vi "test-swerve-drive-kinematics-03.vi"() -> (3 "Test Passed":bool)   [LabVIEW 2019]
uses:
  <vilib>/Rock Robotics/WPI/ThirdParty/JAS_Junk/TrajLib/SWERVE_DRIVE_MODULE_STATE.ctl
  <vilib>/Rock Robotics/WPI/ThirdParty/JAS_Junk/TrajLib/ROTATION2D.ctl
  <vilib>/Rock Robotics/WPI/ThirdParty/JAS_Junk/TrajLib/Trajectory_Library.lvlib
panel:
  out "ModuleStates":T1[](array[typedef]) {"Angle"."SIN" format="%13.4f"; "Angle"."COS" format="%13.4f"; "Angle"."VALUE" format="%13.4f"}
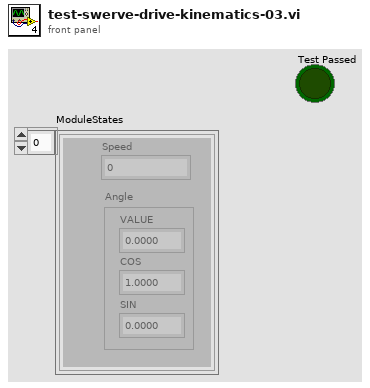
[diagram p1: front panel]
types:
  T1 = typedef "Trajectory_Library.lvlib/SWERVE_DRIVE_MODULE_STATE.ctl" = cluster{"Speed":dbl, "Angle":T2}
  T2 = typedef "Trajectory_Library.lvlib/ROTATION2D.ctl" = cluster{"VALUE":dbl, "COS":dbl, "SIN":dbl}
  T3 = typedef "Trajectory_Library.lvlib/TRANSLATION2D.ctl" = cluster{"X":dbl, "Y":dbl}
  T4 = typedef "Trajectory_Library.lvlib/SWERVE_DRIVE_KINEMATICS.ctl" = cluster{"NumModules":i32, "InverseKinematics":T5, "ForwardKinematics":T5, "Modules":T3[], "PrevCoR":T3}
  T5 = typedef "NI_Matrix.lvlib/RealMatrix.ctl" = dbl[][]
  T6 = typedef "Trajectory_Library.lvlib/CHASSIS_SPEEDS.ctl" = cluster{"vX":dbl, "vY":dbl, "vOmega":dbl}
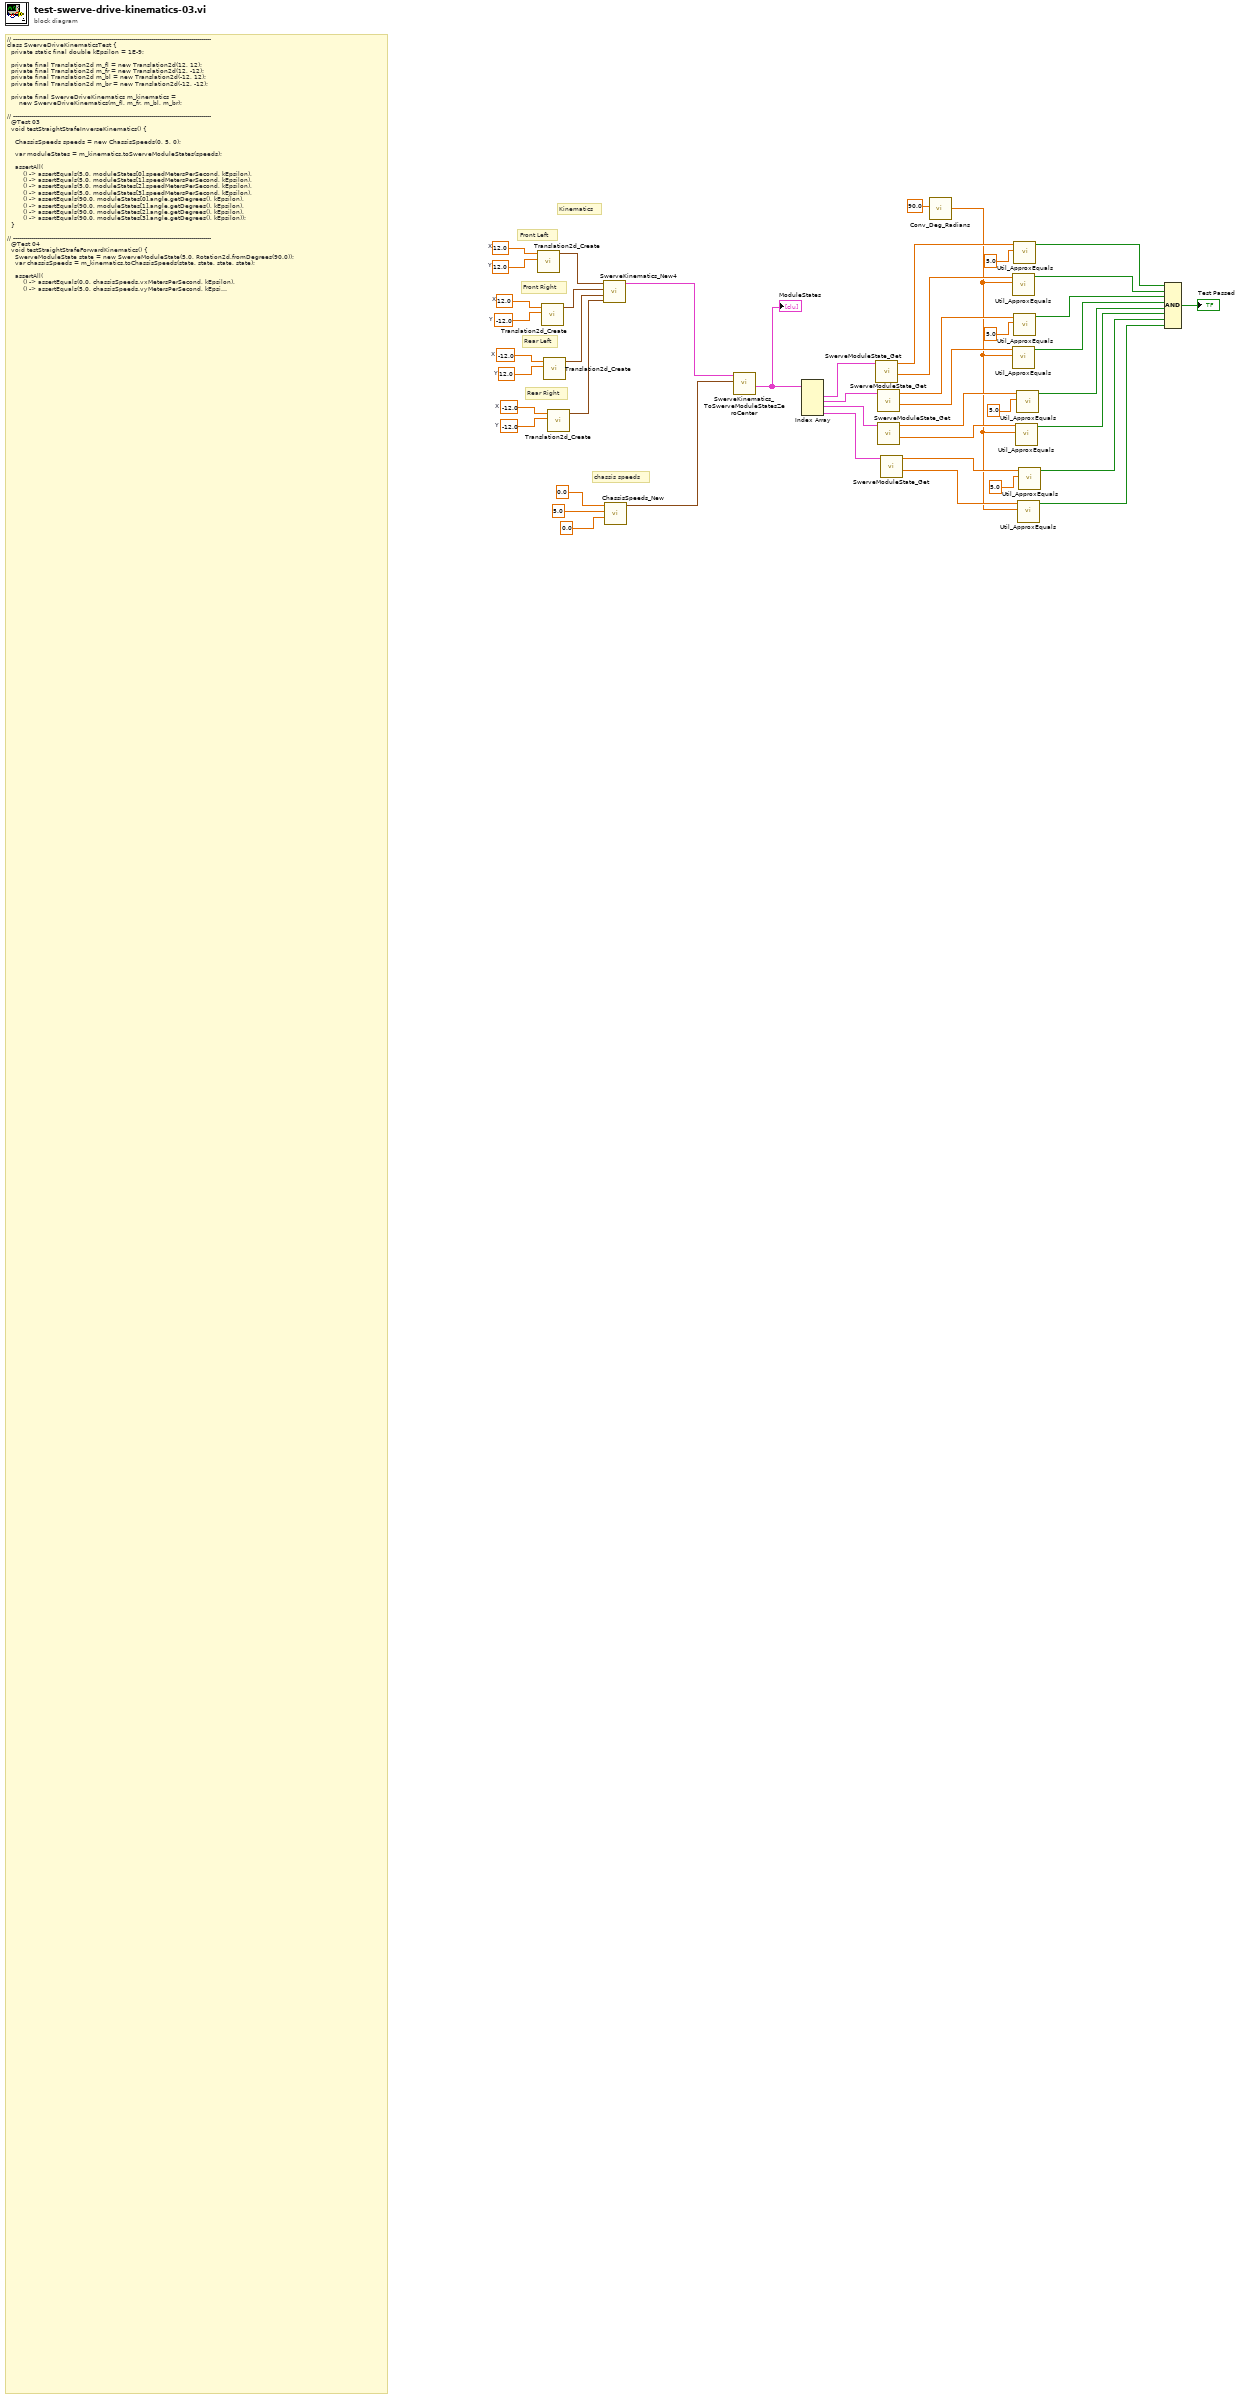
[diagram p0: block diagram]
diagram:
  w38 = -12.0  # X
  w37 = -12.0  # Y
  w36 = -12.0  # X
  w35 = 12.0  # Y
  w34 = 12.0  # X
  w33 = -12.0  # Y
  w32 = 12.0  # X
  w31 = 12.0  # Y
  # "Kinematics"
  # "Rear Right"
  # "Rear Left"
  # "Front Right"
  # "Front Left"
  # "chassis speeds"
  # "// ---------------------------------------------------------------------------------------------------\nclass SwerveDriveKinematicsTest {\n  private static final double kEpsilon = 1E-9;\n\n  private final Translation2d m_fl = new Translation2d(12, 12);\n  private final Translation2d m_fr = new Translation2d(12, -12);\n  private final Translation2d m_bl = new Translation2d(-12, 12);\n  private final Translation2d m_br = new Translation2d(-12, -12);\n\n  private final SwerveDriveKinematics m_kinematics =\n      new SwerveDriveKinematics(m_fl, m_fr, m_bl, m_br);\n\n// ---------------------------------------------------------------------------------------------------\n  @Test 03\n  void testStraightStrafeInverseKinematics() {\n\n    ChassisSpeeds speeds = new ChassisSpeeds(0, 5, 0);\n\n    var moduleStates = m_kinematics.toSwerveModuleStates(speeds);\n\n    assertAll(\n        () -> assertEquals(5.0, moduleStates[0].speedMetersPerSecond, kEpsilon),\n        () -> assertEquals(5.0, moduleStates[1].speedMetersPerSecond, kEpsilon),\n        () -> assertEquals(5.0, moduleStates[2].speedMetersPerSecond, kEpsilon),\n        () -> assertEquals(5.0, moduleStates[3].speedMetersPerSecond, kEpsilon),\n        () -> assertEquals(90.0, moduleStates[0].angle.getDegrees(), kEpsilon),\n        () -> assertEquals(90.0, moduleStates[1].angle.getDegrees(), kEpsilon),\n        () -> assertEquals(90.0, moduleStates[2].angle.getDegrees(), kEpsilon),\n        () -> assertEquals(90.0, moduleStates[3].angle.getDegrees(), kEpsilon));\n  }\n\n// ---------------------------------------------------------------------------------------------------\n  @Test 04\n  void testStraightStrafeForwardKinematics() {\n    SwerveModuleState state = new SwerveModuleState(5.0, Rotation2d.fromDegrees(90.0));\n    var chassisSpeeds = m_kinematics.toChassisSpeeds(state, state, state, state);\n\n    assertAll(\n        () -> assertEquals(0.0, chassisSpeeds.vxMetersPerSecond, kEpsilon),\n        () -> assertEquals(5.0, chassisSpeeds.vyMetersPerSecond, kEpsilon),\n        () -> assertEquals(0.0, chassisSpeeds.omegaRadiansPerSecond, kEpsilon));\n  }\n\n// ---------------------------------------------------------------------------------------------------\n  @Test 05\n  void testTurnInPlaceInverseKinematics() {\n    ChassisSpeeds speeds = new ChassisSpeeds(0, 0, 2 * Math.PI);\n    var moduleStates = m_kinematics.toSwerveModuleStates(speeds);\n\n    /*\n    The circumference of the wheels about the COR is pi * diameter, or 2 * pi * radius\n    the radius is the sqrt(12^2in + 12^2in), or 16.9706in, so the circumference the wheels\n    trace out is 106.629190516in. since we want our robot to rotate at 1 rotation per second,\n    our wheels must trace out 1 rotation (or 106.63 inches) per second.\n      */\n\n    assertAll(\n        () -> assertEquals(106.63, moduleStates[0].speedMetersPerSecond, 0.1),\n        () -> assertEquals(106.63, moduleStates[1].speedMetersPerSecond, 0.1),\n        () -> assertEquals(106.63, moduleStates[2].speedMetersPerSecond, 0.1),\n        () -> assertEquals(106.63, moduleStates[3].speedMetersPerSecond, 0.1),\n        () -> assertEquals(135.0, moduleStates[0].angle.getDegrees(), kEpsilon),\n        () -> assertEquals(45.0, moduleStates[1].angle.getDegrees(), kEpsilon),\n        () -> assertEquals(-135.0, moduleStates[2].angle.getDegrees(), kEpsilon),\n        () -> assertEquals(-45.0, moduleStates[3].angle.getDegrees(), kEpsilon));\n  }\n\n// ---------------------------------------------------------------------------------------------------\n  @Test 06\n  void testTurnInPlaceForwardKinematics() {\n    SwerveModuleState flState = new SwerveModuleState(106.629, Rotation2d.fromDegrees(135));\n    SwerveModuleState frState = new SwerveModuleState(106.629, Rotation2d.fromDegrees(45));\n    SwerveModuleState blState = new SwerveModuleState(106.629, Rotation2d.fromDegrees(-135));\n    SwerveModuleState brState = new SwerveModuleState(106.629, Rotation2d.fromDegrees(-45));\n\n    var chassisSpeeds = m_kinematics.toChassisSpeeds(flState, frState, blState, brState);\n\n    assertAll(\n        () -> assertEquals(0.0, chassisSpeeds.vxMetersPerSecond, kEpsilon),\n        () -> assertEquals(0.0, chassisSpeeds.vyMetersPerSecond, kEpsilon),\n        () -> assertEquals(2 * Math.PI, chassisSpeeds.omegaRadiansPerSecond, 0.1));\n  }\n\n// ---------------------------------------------------------------------------------------------------\n  @Test 07\n  void testOffCenterCORRotationInverseKinematics() {\n    ChassisSpeeds speeds = new ChassisSpeeds(0, 0, 2 * Math.PI);\n    var moduleStates = m_kinematics.toSwerveModuleStates(speeds, m_fl);\n\n    /*\n    This one is a bit trickier. Because we are rotating about the front-left wheel,\n    it should be parked at 0 degrees and 0 speed. The front-right and back-left wheels both travel\n    an arc with radius 24 (and circumference 150.796), and the back-right wheel travels an arc with\n    radius sqrt(24^2 + 24^2) and circumference 213.2584. As for angles, the front-right wheel\n    should be pointing straight forward, the back-left wheel should be pointing straight right,\n    and the back-right wheel should be at a -45 degree angle\n    */\n\n    assertAll(\n        () -> assertEquals(0.0, moduleStates[0].speedMetersPerSecond, 0.1),\n        () -> assertEquals(150.796, moduleStates[1].speedMetersPerSecond, 0.1),\n        () -> assertEquals(150.796, moduleStates[2].speedMetersPerSecond, 0.1),\n        () -> assertEquals(213.258, moduleStates[3].speedMetersPerSecond, 0.1),\n        () -> assertEquals(0.0, moduleStates[0].angle.getDegrees(), kEpsilon),\n        () -> assertEquals(0.0, moduleStates[1].angle.getDegrees(), kEpsilon),\n        () -> assertEquals(-90.0, moduleStates[2].angle.getDegrees(), kEpsilon),\n        () -> assertEquals(-45.0, moduleStates[3].angle.getDegrees(), kEpsilon));\n  }\n\n// ---------------------------------------------------------------------------------------------------\n  @Test 08\n  void testOffCenterCORRotationForwardKinematics() {\n    SwerveModuleState flState = new SwerveModuleState(0.0, Rotation2d.fromDegrees(0.0));\n    SwerveModuleState frState = new SwerveModuleState(150.796, Rotation2d.fromDegrees(0.0));\n    SwerveModuleState blState = new SwerveModuleState(150.796, Rotation2d.fromDegrees(-90));\n    SwerveModuleState brState = new SwerveModuleState(213.258, Rotation2d.fromDegrees(-45));\n\n    var chassisSpeeds = m_kinematics.toChassisSpeeds(flState, frState, blState, brState);\n\n    /*\n    We already know that our omega should be 2pi from the previous test. Next, we need to determine\n    the vx and vy of our chassis center. Because our COR is at a 45 degree angle from the center,\n    we know that vx and vy must be the same. Furthermore, we know that the center of mass makes\n    a full revolution about the center of revolution once every second. Therefore, the center of\n    mass must be moving at 106.629in/sec. Recalling that the ratios of a 45/45/90 triagle are\n    1:sqrt(2)/2:sqrt(2)/2, we find that the COM vx is -75.398, and vy is 75.398.\n    */\n\n    assertAll(\n        () -> assertEquals(75.398, chassisSpeeds.vxMetersPerSecond, 0.1),\n        () -> assertEquals(-75.398, chassisSpeeds.vyMetersPerSecond, 0.1),\n        () -> assertEquals(2 * Math.PI, chassisSpeeds.omegaRadiansPerSecond, 0.1));\n  }\n\n  private void assertModuleState(\n      SwerveModuleState expected, SwerveModuleState actual, SwerveModuleState tolerance) {\n    assertAll(\n        () ->\n            assertEquals(\n                expected.speedMetersPerSecond,\n                actual.speedMetersPerSecond,\n                tolerance.speedMetersPerSecond),\n        () ->\n            assertEquals(\n                expected.angle.getDegrees(),\n                actual.angle.getDegrees(),\n                tolerance.angle.getDegrees()));\n  }\n\n// ---------------------------------------------------------------------------------------------------\n  /**\n   * Test the rotation of the robot about a non-central point with both linear and angular\n   * velocities.\n   */\n  @Test 09\n  void testOffCenterCORRotationAndTranslationInverseKinematics() {\n    ChassisSpeeds speeds = new ChassisSpeeds(0.0, 3.0, 1.5);\n    var moduleStates = m_kinematics.toSwerveModuleStates(speeds, new Translation2d(24, 0));\n\n    // By equation (13.14) from state-space guide, our wheels/angles will be as follows,\n    // (+-1 degree or speed):\n    SwerveModuleState[] expectedStates =\n        new SwerveModuleState[] {\n          new SwerveModuleState(23.43, Rotation2d.fromDegrees(-140.19)),\n          new SwerveModuleState(23.43, Rotation2d.fromDegrees(-39.81)),\n          new SwerveModuleState(54.08, Rotation2d.fromDegrees(-109.44)),\n          new SwerveModuleState(54.08, Rotation2d.fromDegrees(-70.56))\n        };\n    var stateTolerance = new SwerveModuleState(0.1, Rotation2d.fromDegrees(0.1));\n\n    for (int i = 0; i < expectedStates.length; i++) {\n      assertModuleState(expectedStates[i], moduleStates[i], stateTolerance);\n    }\n  }\n\n// ---------------------------------------------------------------------------------------------------\n  @Test 10\n  void testOffCenterCORRotationAndTranslationForwardKinematics() {\n    SwerveModuleState flState = new SwerveModuleState(23.43, Rotation2d.fromDegrees(-140.19));\n    SwerveModuleState frState = new SwerveModuleState(23.43, Rotation2d.fromDegrees(-39.81));\n    SwerveModuleState blState = new SwerveModuleState(54.08, Rotation2d.fromDegrees(-109.44));\n    SwerveModuleState brState = new SwerveModuleState(54.08, Rotation2d.fromDegrees(-70.56));\n\n    var chassisSpeeds = m_kinematics.toChassisSpeeds(flState, frState, blState, brState);\n\n    /*\n    From equation (13.17), we know that chassis motion is th dot product of the\n    pseudoinverse of the inverseKinematics matrix (with the center of rotation at\n    (0,0) -- we don't want the motion of the center of rotation, we want it of\n    the center of the robot). These above SwerveModuleStates are known to be from\n    a velocity of [[0][3][1.5]] about (0, 24), and the expected numbers have been\n    calculated using Numpy's linalg.pinv function.\n    */\n\n    assertAll(\n        () -> assertEquals(0.0, chassisSpeeds.vxMetersPerSecond, 0.1),\n        () -> assertEquals(-33.0, chassisSpeeds.vyMetersPerSecond, 0.1),\n        () -> assertEquals(1.5, chassisSpeeds.omegaRadiansPerSecond, 0.1));\n  }\n\n// ---------------------------------------------------------------------------------------------------\n  @Test 11\n  void testNormalize() {\n    SwerveModuleState fl = new SwerveModuleState(5, new Rotation2d());\n    SwerveModuleState fr = new SwerveModuleState(6, new Rotation2d());\n    SwerveModuleState bl = new SwerveModuleState(4, new Rotation2d());\n    SwerveModuleState br = new SwerveModuleState(7, new Rotation2d());\n\n    SwerveModuleState[] arr = {fl, fr, bl, br};\n    SwerveDriveKinematics.normalizeWheelSpeeds(arr, 5.5);\n\n    double factor = 5.5 / 7.0;\n\n    assertAll(\n        () -> assertEquals(5.0 * factor, arr[0].speedMetersPerSecond, kEpsilon),\n        () -> assertEquals(6.0 * factor, arr[1].speedMetersPerSecond, kEpsilon),\n        () -> assertEquals(4.0 * factor, arr[2].speedMetersPerSecond, kEpsilon),\n        () -> assertEquals(7.0 * factor, arr[3].speedMetersPerSecond, kEpsilon));\n  }\n}"
  n1 = call <vilib>:"Translation2d_Create.vi"("Y"=w31, "X"=w32) -> ("TRANSLATION"=w39:T3)  [unwired: 9 in]
  n2 = call <vilib>:"Translation2d_Create.vi"("Y"=w33, "X"=w34) -> ("TRANSLATION"=w40:T3)  [unwired: 9 in]
  n3 = call <vilib>:"Translation2d_Create.vi"("Y"=w35, "X"=w36) -> ("TRANSLATION"=w41:T3)  [unwired: 9 in]
  n4 = call <vilib>:"Translation2d_Create.vi"("Y"=w37, "X"=w38) -> ("TRANSLATION"=w42:T3)  [unwired: 9 in]
  n5 = call <vilib>:"SwerveKinematics_New4.vi"("wheel 3"=w42, "wheel 2"=w41, "wheel 1"=w40, "wheel 0"=w39) -> ("SWERVE_DRIVE_KINEMATICS"=w30:T4)  [unwired: 7 in]
  n6 = call <vilib>:"ChassisSpeeds_New.vi"("vAngular"=0.0, "vY"=5.0, "vX"=0.0) -> ("CHASSIS"=w29:T6)  [unwired: 8 in]
  n7 = call <vilib>:"SwerveKinematics_ToSwerveModuleStatesZeroCenter.vi"("ChassisSpeeds"=w29, "in SWERVE_DRIVE_KINEMATICS"=w30) -> ("ModuleStates"=w28:T1[])  [unwired: 8 in, 1 out]
  "ModuleStates" <- w28
  n8 = Index Array(array=w28) -> (element #1=w27:T1, element #2=w26:T1, element #3=w25:T1, element #4=w24:T1)  [unwired: 4 in]
  n9 = call <vilib>:"SwerveModuleState_Get.vi"("Desired State"=w27) -> ("Angle RADIANS"=w18:dbl, "Speed M/S"=w19:dbl)  [unwired: 9 in]
  n10 = call <vilib>:"SwerveModuleState_Get.vi"("Desired State"=w26) -> ("Angle RADIANS"=w16:dbl, "Speed M/S"=w17:dbl)  [unwired: 9 in]
  n11 = call <vilib>:"SwerveModuleState_Get.vi"("Desired State"=w25) -> ("Angle RADIANS"=w14:dbl, "Speed M/S"=w15:dbl)  [unwired: 9 in]
  n12 = call <vilib>:"SwerveModuleState_Get.vi"("Desired State"=w24) -> ("Angle RADIANS"=w12:dbl, "Speed M/S"=w13:dbl)  [unwired: 9 in]
  n13 = call <vilib>:"Conv_Deg_Radians.vi"("Degress"=90.0) -> ("Radians"=w1:dbl)  [unwired: 10 in]
  n14 = call <vilib>:"Util_ApproxEquals.vi"("Value 2"=w1, "Value 1"=w18) -> ("ApproxEquals"=w10:bool)  [unwired: 9 in]
  n15 = call <vilib>:"Util_ApproxEquals.vi"("Value 2"=w1, "Value 1"=w16) -> ("ApproxEquals"=w8:bool)  [unwired: 9 in]
  n16 = call <vilib>:"Util_ApproxEquals.vi"("Value 2"=5.0, "Value 1"=w19) -> ("ApproxEquals"=w11:bool)  [unwired: 9 in]
  n17 = call <vilib>:"Util_ApproxEquals.vi"("Value 2"=5.0, "Value 1"=w17) -> ("ApproxEquals"=w9:bool)  [unwired: 9 in]
  n18 = call <vilib>:"Util_ApproxEquals.vi"("Value 2"=w1, "Value 1"=w14) -> ("ApproxEquals"=w6:bool)  [unwired: 9 in]
  n19 = call <vilib>:"Util_ApproxEquals.vi"("Value 2"=5.0, "Value 1"=w15) -> ("ApproxEquals"=w7:bool)  [unwired: 9 in]
  n20 = call <vilib>:"Util_ApproxEquals.vi"("Value 2"=w1, "Value 1"=w12) -> ("ApproxEquals"=w4:bool)  [unwired: 9 in]
  n21 = call <vilib>:"Util_ApproxEquals.vi"("Value 2"=5.0, "Value 1"=w13) -> ("ApproxEquals"=w5:bool)  [unwired: 9 in]
  n22 = Compound Arithmetic op=AND(w11, w10, w9, w8, w7, w6, w5, w4) -> (→"Test Passed":bool)
